vi "Record_Video.vi"(8 "error in (no error)":errorcluster, 10 "Data In":T4 {"Frame Data"."Image Type" items=["Grayscale (U8)", "Grayscale (I16)", "Grayscale (SGL)", "Complex (CSG)", "RGB (U32)", "HSL (U32)", "RGB (U64)", "Grayscale (U16)"]}, 11 "Recording Data In":T1) -> (0 "error out":errorcluster, 3 "Recording Data Out":T1)   [LabVIEW 2017, in "ImageAcquisitionLibrary.lvlib"]
uses:
  ImageAcquisitionLibrary.lvlib
  Acquisition/AcquireData.ctl
  RecordingData.ctl
  <vilib>/vision/Image Controls.llb/IMAQ Image.ctl
  <vilib>/vision/Avi.llb/IMAQ AVI2 Refnum.ctl
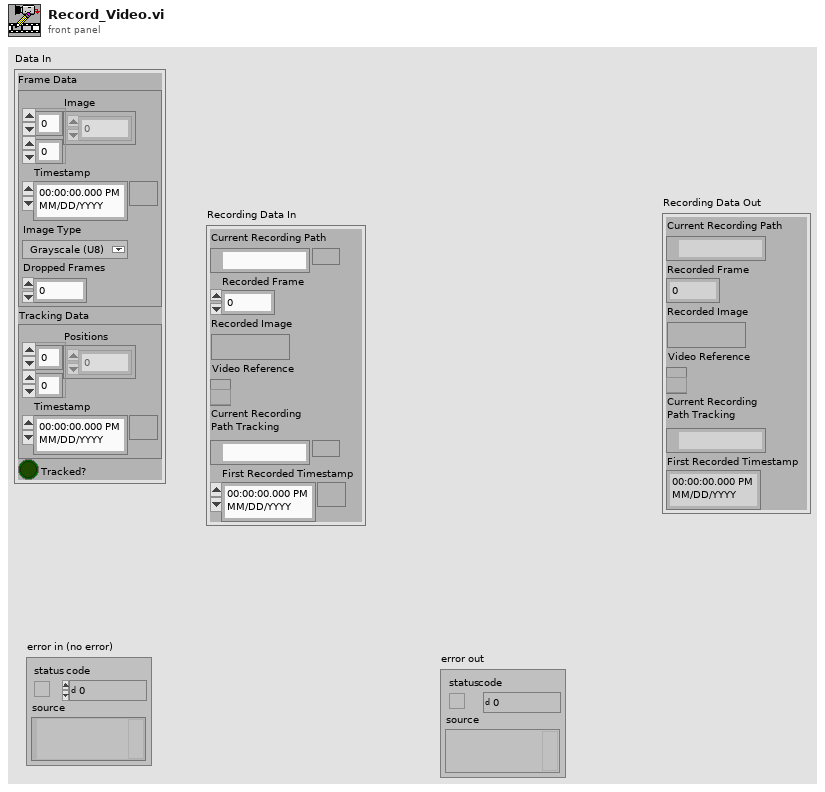
[diagram p1: front panel]
types:
  T1 = typedef "ImageAcquisitionLibrary.lvlib/RecordingData.ctl" = cluster{"Current Recording Path":path, "Recorded Frame":i32, "Recorded Image":T2, "Video Reference":T3, "Current Recording \nPath Tracking":path, "First Recorded Timestamp":timestamp}
  T2 = typedef "IMAQ Image.ctl" = refnum<image>
  T3 = typedef "IMAQ AVI2 Refnum.ctl" = refnum<k20>
  T4 = typedef "ImageAcquisitionLibrary.lvlib/AcquireData.ctl" = cluster{"Frame Data":cluster{"Image":u32[][], "Timestamp":timestamp, "Image Type":T5, "Dropped Frames":u32}, "Tracking Data":cluster{"Positions":dbl[][], "Timestamp":timestamp}, "Tracked?":bool}
  T5 = typedef "Image Type" = u32
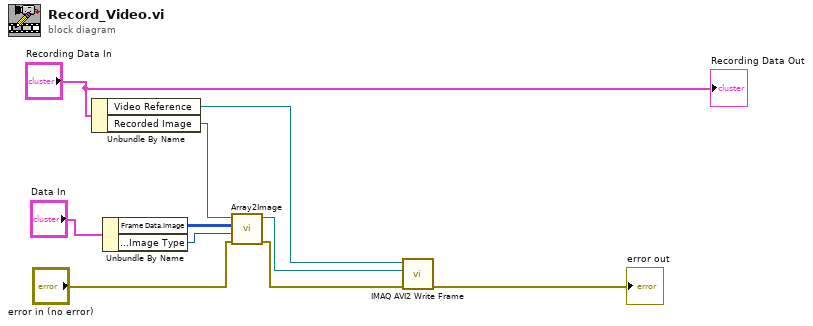
[diagram p0: block diagram]
diagram:
  n1 = Unbundle By Name("Recording Data In") -> ("Video Reference"=w9:T3, "Recorded Image"=w6:T2)
  n2 = Unbundle By Name("Data In") -> ("Frame Data.Image"=w3:u32[][], "Frame Data.Image Type"=w2:T5)
  n3 = call "Array2Image.vi"("error in (no error)"="error in (no error)", "Image Type"=w2, "Image Pixels (U32)"=w3, "Image 2"=w6) -> ("error out"=w4:errorcluster, "Image"=w1:T2)  [unwired: 6 in]
  n4 = call "IMAQ AVI2 Write Frame"("error in (no error)"=w4, "Image"=w1, "AVI Refnum"=w9) -> ("error out"=→"error out":errorcluster)  [unwired: 6 in, 2 out]
  "Recording Data Out" <- "Recording Data In"
